vi "Read Active Frame.vi"(9 "DiagramDisable in":refnum<class "DiagramDisable.lvclass">) -> (3 "DiagramDisable out":refnum<class "DiagramDisable.lvclass">, 4 "Active Frame":i16)   [LabVIEW 2014, in "DiagramDisable.lvclass"]
uses:
  DiagramDisable.lvclass
  DiagramDisable.lvclass/DiagramDisable.ctl
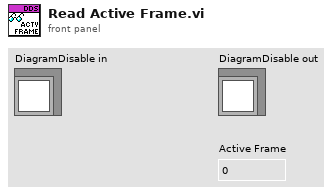
[diagram p1: front panel]
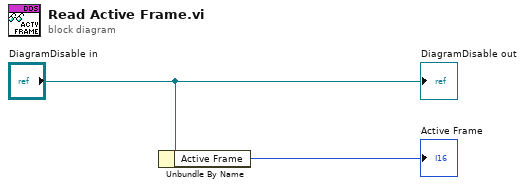
[diagram p0: block diagram]
diagram:
  n1 = Unbundle By Name("DiagramDisable in") -> ("Active Frame"=→"Active Frame":i16)
  "DiagramDisable out" <- "DiagramDisable in"
